vi "Rotation Matrix to Roll Pitch Yaw.vi"(1 "rotation matrix":T1) -> (0 "angles":cluster{"roll":dbl, "pitch":dbl, "yaw":dbl})   [LabVIEW 2021]
doc: "This VI transforms rotation matrix to roll pitch yaw."
uses:
  <vilib>/Analysis/Matrix/Datatypes/RealMatrix.ctl
  <vilib>/Analysis/Matrix/NI_Matrix.lvlib
panel:
  # "This VI transforms rotation matrix to roll pitch yaw."
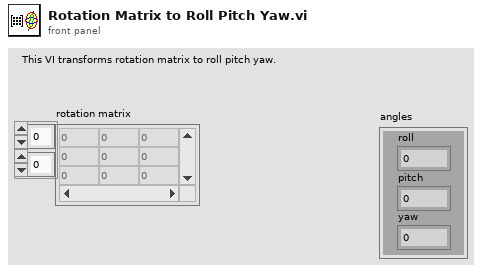
[diagram p1: front panel]
types:
  T1 = typedef "NI_Matrix.lvlib/RealMatrix.ctl" = dbl[][]
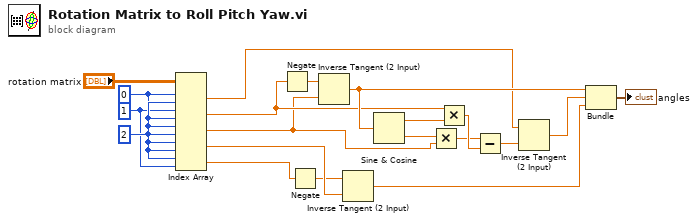
[diagram p0: block diagram]
diagram:
  w1 = 1 ("index (row)")
  w3 = 2 ("index (col)")
  w2 = 0 ("index (row)")
  n1 = Index Array(array="rotation matrix", index (row) #1=w2, index (col) #1=w3, index (row) #2=w1, index (col) #2=w3, index (row) #3=w3, index (col) #3=w3, index (row) #4=w2, index (col) #4=w2, index (row) #5=w2, index (col) #5=w1) -> (element #1=w7:dbl, element #2=w11:dbl, element #3=w4:dbl, element #4=w15:dbl, element #5=w19:dbl)
  n2 = Negate(x=w11) -> (-x=w16:dbl)
  n3 = Negate(x=w19) -> (-x=w14:dbl)
  n4 = Inverse Tangent (2 Input)(1:w4, 2:w16) -> (0:w13:dbl)
  n5 = Inverse Tangent (2 Input)(1:w15, 2:w14) -> (0:w18:dbl)
  n6 = Sine & Cosine(0:w13) -> (1:w12:dbl, 2:w5:dbl)
  n7 = Multiply(x=w5, y=w4) -> (x*y=w9:dbl)
  n8 = Multiply(x=w11, y=w12) -> (x*y=w10:dbl)
  n9 = Subtract(x=w9, y=w10) -> (x-y=w6:dbl)
  n10 = Inverse Tangent (2 Input)(1:w6, 2:w7) -> (0:w17:dbl)
  n11 = Bundle(w13, w17, w18) -> (→"angles":cluster{dbl, dbl, dbl})  [unwired: 1 in]
